vi "Button Test State.vi"(0 "GEA2 Reference Out in":refnum<k24>, 5 "Queue in":refnum<queue>, 9 "Test Results in":T1, 11 "error in (no error)":errorcluster) -> (4 ".NET Refnum out":refnum<k24>, 10 "Test Results out":T1, 15 "error out":errorcluster)   [LabVIEW 2016]
doc: "This VI performs the button press test state."
uses:
  controls/Test Results.ctl
  C:/Program Files (x86)/National Instruments/LabVIEW 2016/examples/Design Patterns/Queued Message Handler/support/QMH Fundamentals - Message Cluster.ctl
  C:/Automation/DLLs/PC Dot Net/GeaCommunication.dll
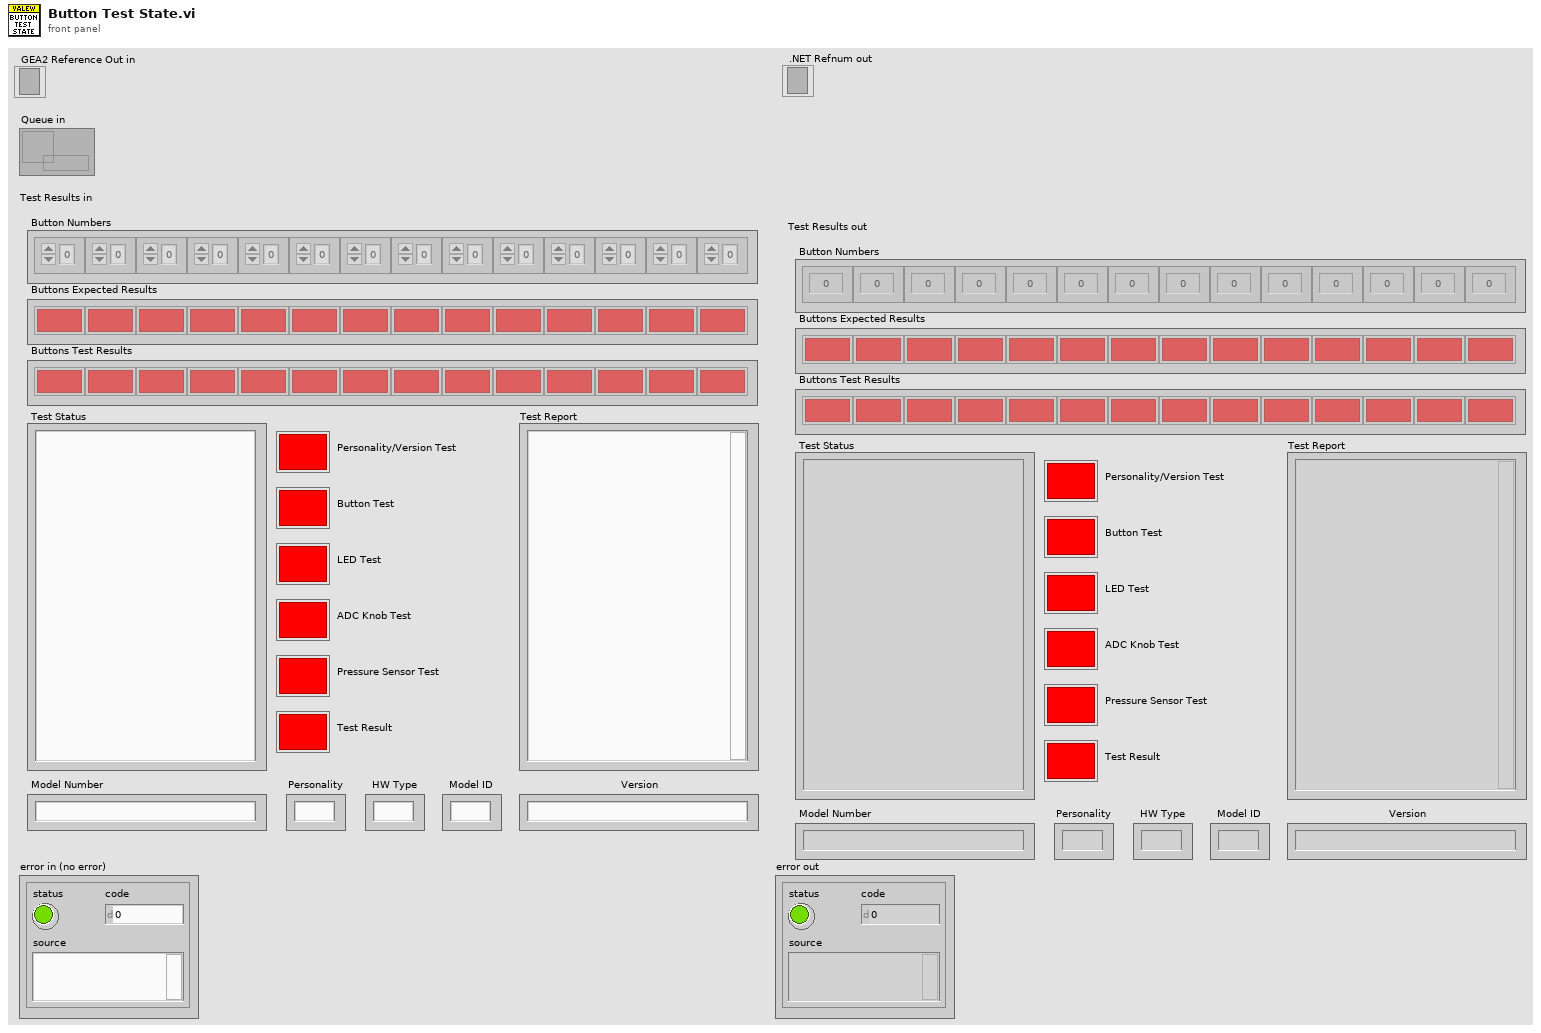
[diagram p1: front panel]
types:
  T1 = typedef "Test Results.ctl" = cluster{"Test Status":string, "Personality/Version Test ":bool, "Test Report":string, "Model Number":string, "Button Numbers":i32[], "Buttons Test Results":bool[], "Buttons Expected Results":bool[], "Model ID":string, "Personality":string, "HW Type":string, "Version":string, "Button Test":bool, "LED Test":bool, "ADC Knob Test":bool, "Pressure Sensor Test":bool, "Test Result":bool}
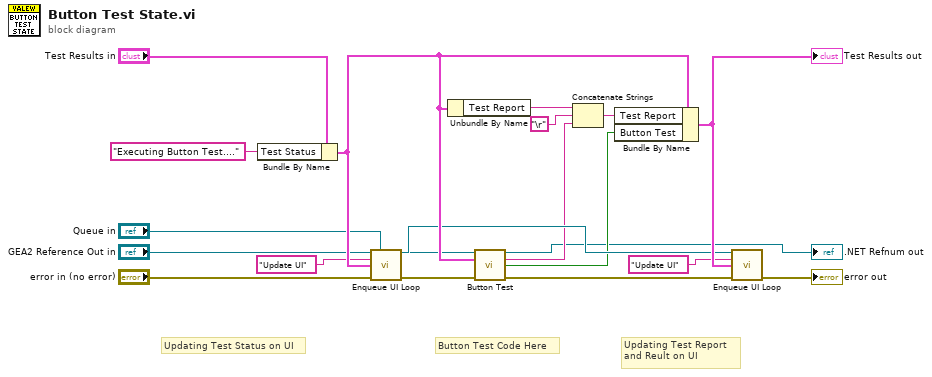
[diagram p0: block diagram]
diagram:
  # "Updating Test Report \nand Reult on UI"
  # "Button Test Code Here"
  # "Updating Test Status on UI"
  n1 = Bundle By Name(cluster="Test Results in", "Test Status"="Executing Button Test....") -> (w19:T1)
  n2 = call "Enqueue UI Loop.vi"("UI Que In"="Queue in", "Message"="Update UI", "Test Results"=w19, "error in (no error)"="error in (no error)") -> ("UI Queue Out"=w16:refnum<queue>, "error out"=w11:errorcluster)  [unwired: 10 in]
  n3 = Unbundle By Name(w19) -> ("Test Report"=w4:string)
  n4 = call "Button Test.vi"("GEA2 Reference In"="GEA2 Reference Out in", "Test Results In"=w19, "Error In"=w11) -> ("GEA2 Reference Out"=→".NET Refnum out":refnum<k24>, "Report Text"=w6:string, "Pass/Fail?"=w3:bool, "Error Out"=w14:errorcluster)  [unwired: 9 in]
  n5 = Concatenate Strings(w4, "\r", w6) -> (w7:string)
  n6 = Bundle By Name(cluster=w19, "Test Report"=w7, "Button Test"=w3) -> (w18:T1)
  "Test Results out" <- w18
  n7 = call "Enqueue UI Loop.vi"("UI Que In"=w16, "Message"="Update UI", "Test Results"=w18, "error in (no error)"=w14) -> ("error out"=→"error out":errorcluster)  [unwired: 10 in, 1 out]
